vi "GetBufferSize.vi"(8 "error in (no error)":errorcluster, 11 "Handle":refnum<data-value>) -> (0 "error out":errorcluster, 3 "Size":i32)   [LabVIEW 2020, in "Buffer.lvclass"]
uses:
  Buffer.lvclass
  Buffer.lvclass/Buffer.ctl
  bin/gindustrialcam_32-1.dll
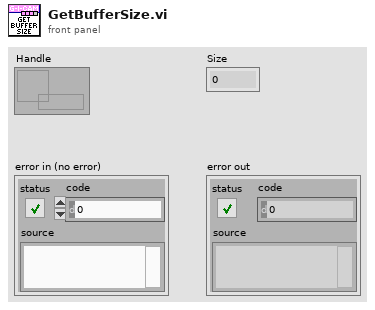
[diagram p1: front panel]
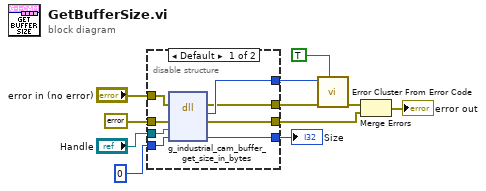
[diagram p0: block diagram]
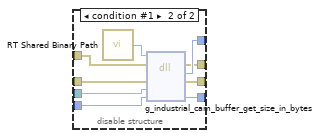
[diagram p2: hidden frame]
diagram:
  n1 = disable-structure shown="Default" {
    disable-tunnel: [w19 w28] -> w11
    disable-tunnel: 0 ("size") -> [w18 w27]
    disable-tunnel: "Handle" -> [w17 w26]
    disable-tunnel: "error in (no error)" -> [w16 w25]
    disable-tunnel: errorcluster {"status"=FALSE, "code"=0, "source"=""} ("error constant") -> [w15 w24]
    disable-tunnel: [w14 w23] -> w4
    disable-tunnel: [w13 w22] -> w2
    disable-tunnel: [w12 w21] -> w1
    frame condition #0 (active) {
      n2 = dll-call lib="C:/serenial/lib/g-industrial-camera/LabVIEW/g_industrial_cam/bin/gindustrialcam_*-1.*" fn="g_industrial_cam_buffer_get_size_in_bytes"(error in=w16, "err"=w15, "edvr"=w17, "size"=w18) -> (error out=w12:errorcluster, "Mg_Error"=w13:i32, "err"=w14:errorcluster, "size"=w19:i32)  [unwired: 3 in, 1 out]
    }
    frame condition #1 {
      n3 = call "RT Shared Binary Path.vi"() -> ("Path"=w20:path)
      n4 = dll-call lib="C:/serenial/lib/g-industrial-camera/LabVIEW/g_industrial_cam/bin/gindustrialcam_*-1.*" fn="g_industrial_cam_buffer_get_size_in_bytes"(path in=w20, error in=w25, "err"=w24, "edvr"=w26, "size"=w27) -> (error out=w21:errorcluster, "Mg_Error"=w22:i32, "err"=w23:errorcluster, "size"=w28:i32)  [unwired: 2 in, 1 out]
    }
  }
  "Size" <- w11
  n5 = call <vilib>:"Error Cluster From Error Code.vi"("show call chain? (False)"=TRUE, "error in (no error)"=w1, "error code (0)"=w2) -> ("error out"=w3:errorcluster)  [unwired: 6 in]
  n6 = Merge Errors(w3, w4) -> (→"error out":errorcluster)
